vi "Read ILCADC.vi"(11 "ILC in":refnum<class "ILC.lvclass">) -> (2 "ILC ADC":T1={"Reference Voltage Vref"=0.0, "Nominal Input Range in Counts"=128, "Preamplifier Gain"=0, "Conversion Settling Cycles"=0} {"Conversion Settling Cycles" min=1; "Preamplifier Gain" min=1; "Nominal Input Range in Counts" min=128; "Reference Voltage Vref" min=-10.0 max=10.0 format="%.3f"}, 3 "ILC out":refnum<class "ILC.lvclass">)   [LabVIEW 2015, in "ILCCommon.lvlib" / "ILC.lvclass"]
uses:
  <userlib>/Common/ILC/ILC/ILC.lvclass
  <userlib>/Common/ILC/Configuration/ILCADC.ctl
  <userlib>/Common/ILC/ILC/ILC.lvclass/ILC.ctl
  <userlib>/Common/ILC/Configuration/ILCConfiguration.lvlib
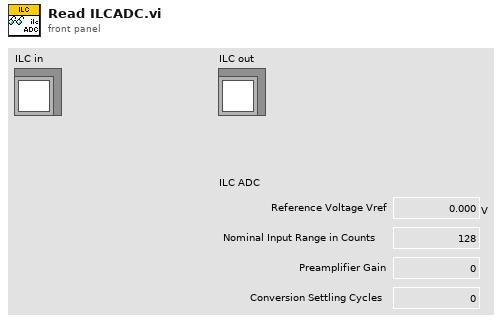
[diagram p1: front panel]
types:
  T1 = typedef "ILCCommon.lvlib/ILCConfiguration.lvlib/ILCADC.ctl" = cluster{"Reference Voltage Vref":dbl[unit], "Nominal Input Range in Counts":u32, "Preamplifier Gain":u8, "Conversion Settling Cycles":u16}
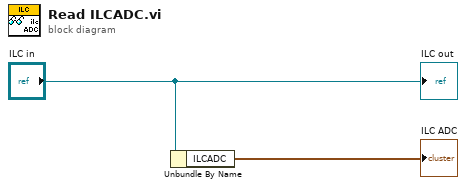
[diagram p0: block diagram]
diagram:
  n1 = Unbundle By Name("ILC in") -> ("ILCADC"=→"ILC ADC":T1)
  "ILC out" <- "ILC in"
